vi "Absolute Value - RM.vi"(1 "Real Matrix A":T1) -> (0 "|A|":T1)   [LabVIEW 2014, in "NI_Matrix.lvlib"]
doc: "Returns the absolute value of the input."
uses:
  NI_Matrix.lvlib
  RealMatrix.ctl
  Array To Matrix - RA2.vi
  Matrix To Array - RM.vi
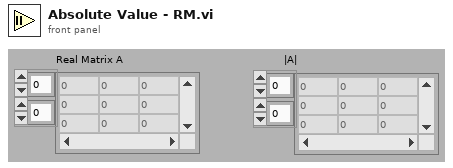
[diagram p1: front panel]
types:
  T1 = typedef "NI_Matrix.lvlib/RealMatrix.ctl" = dbl[][]
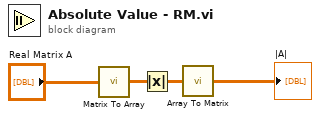
[diagram p0: block diagram]
diagram:
  n1 = call-poly "Matrix To Array.vi"("Real Matrix"="Real Matrix A") -> ("Real 2D Array"=w4:dbl[][])
  n2 = Absolute Value(x=w4) -> (abs(x)=w2:dbl[][])
  n3 = call-poly "Array To Matrix.vi"("Real 2D Array"=w2) -> ("Real Matrix"=→"|A|":T1)
